vi "S7Com_OPEN(SubVI).vi"(6 "timeout ms":i32=25000, 8 "error in (no error)":errorcluster, 9 "PLC type":enum16{"S7-300", "S7-1200"}(ring), 10 "remote port":u16=102, 11 "remote address":string) -> (0 "error out":errorcluster, 1 "PDU Response":T1 format="X%02x", 2 "Connection Confirm CC":T1 format="X%02x", 3 "connection ID out":refnum<k5>, 5 "Error":bool)   [LabVIEW 2019]
doc: "Opens an S7 Connection with a PLC."
uses:
  S7Com_HexByteArray.ctl
  S7Com_HexByte.ctl
panel:
  in  "Connection request CR\nS7-1200":T1=[17, 224, 0, 0, 0, 1, 0, 192, 1, 9, 193, 2, 75, 84, 194, 2, 3, 0] format="X%02x"
  in  "Connection Request CR\nS7-300":T1=[17, 224, 0, 0, 0, 1, 0, 193, 2, 16, 0, 194, 2, 1, 2, 192, 1, 9] format="X%02x"
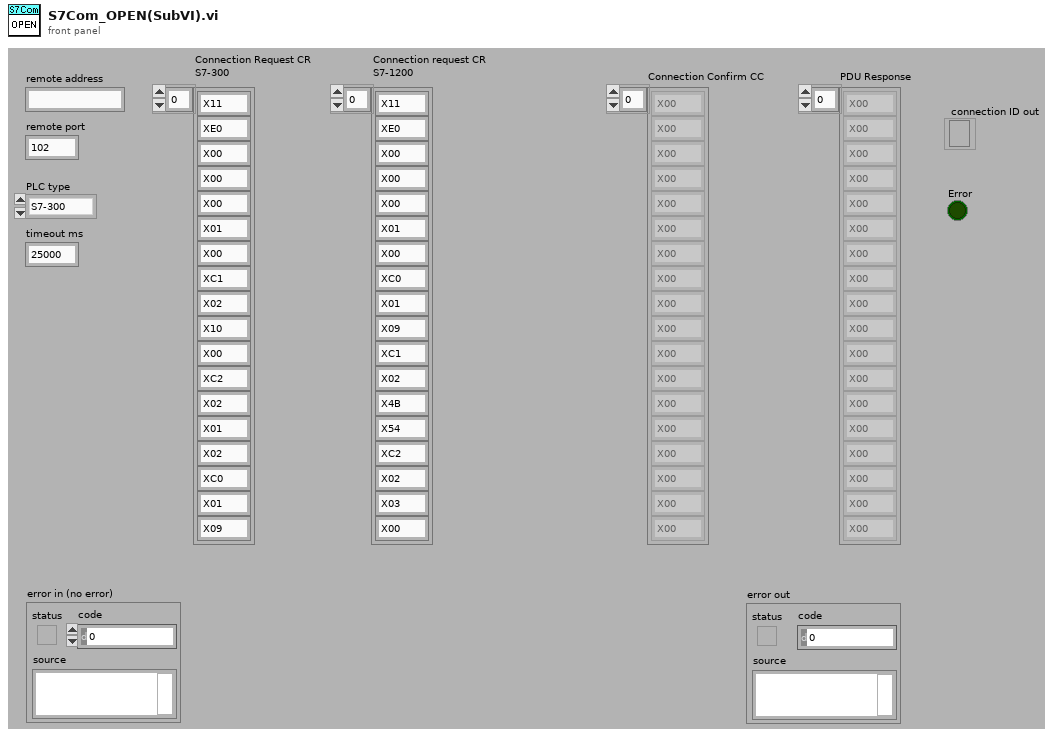
[diagram p1: front panel]
types:
  T1 = typedef "S7Com_HexByteArray.ctl" = T2[]
  T2 = typedef "S7Com_HexByte.ctl" = u8
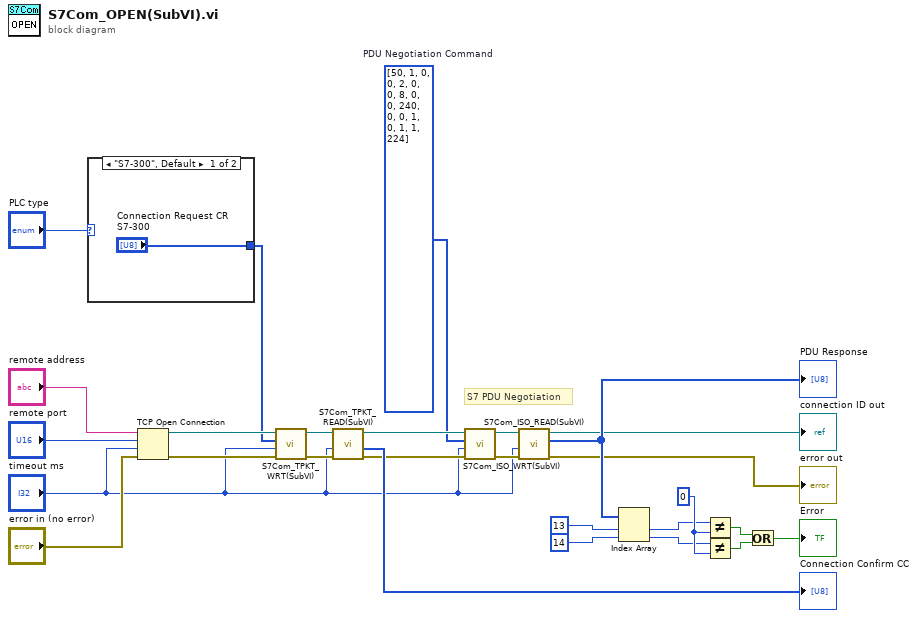
[diagram p0: block diagram]
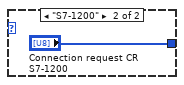
[diagram p2: hidden frame]
diagram:
  w4 = T1 [50, 1, 0, 0, 2, 0, 0, 8, 0, 0, 240, 0, 0, 1, 0, 1, 1, 224]  # PDU Negotiation Command
  w26 = u8 0
  # "S7 PDU Negotiation"
  n1 = case shown="\"S7-300\", Default" "PLC type" {
    tunnel: ["Connection Request CR\nS7-300" "Connection request CR\nS7-1200"] -> w1
    frame "S7-300", Default {
    }
    frame "S7-1200" {
    }
  }
  n2 = TCP Open Connection(address="remote address", remote port or service name="remote port", timeout ms (60000)="timeout ms", error in (no error)="error in (no error)") -> (connection ID=w16:refnum<k5>, error out=w7:errorcluster)  [unwired: 1 out]
  n3 = call "S7Com_TPKT_WRT(SubVI).vi"("error in"=w7, "timeout ms"="timeout ms", "TPDU_In"=w1, "connection ID in"=w16) -> ("error out"=w15:errorcluster, "connection ID out"=w14:refnum<k5>)  [unwired: 2 out]
  n4 = call "S7Com_TPKT_READ(SubVI).vi"("error in"=w15, "timeout ms (25000)"="timeout ms", "connection ID in"=w14) -> ("error out"=w6:errorcluster, "TPDU Data"=→"Connection Confirm CC":T1, "connection ID out"=w17:refnum<k5>)  [unwired: 2 out]
  n5 = call "S7Com_ISO_WRT(SubVI).vi"("error in"=w6, "timeout ms (25000)"="timeout ms", "TPDU_In"=w4, "connection ID in"=w17) -> ("error out"=w12:errorcluster, "connection ID out"=w13:refnum<k5>)  [unwired: 2 out]
  n6 = call "S7Com_ISO_READ(SubVI).vi"("error in"=w12, "timeout ms (25000)"="timeout ms", "connection ID in"=w13) -> ("error out"=→"error out":errorcluster, "TPDU Data"=w19:T1, "connection ID out"=→"connection ID out":refnum<k5>)  [unwired: 2 out]
  "PDU Response" <- w19
  n7 = Index Array(array=w19, index #1=13, index #2=14) -> (element #1=w24:T2, element #2=w25:T2)
  n8 = Not Equal?(x=w24, y=w26) -> (x != y?=w22:bool)
  n9 = Not Equal?(x=w25, y=w26) -> (x != y?=w23:bool)
  n10 = Or(x=w22, y=w23) -> (x .or. y?=→"Error":bool)
